vi "Auton - Center Shoot.vi"(10 "Alliance":T1, 11 "Auton States":T2=enum."Reset Encoders") -> ()   [LabVIEW 2016]
uses:
  Auton - Center Shoot States.ctl
  <vilib>/Rock Robotics/WPI/DriverStation/WPI_DriverStationAllianceInfo.ctl
  Robot Values.vi
panel:
  in  "Move To Boiler SP":dbl
  in  "Red - Turn  to Boiler SP":dbl
  in  "Blue - Turn  to Boiler SP":dbl
  in  "Move Toward Boiler SP":dbl
  in  "Red - Turn to Continue  SP":dbl format="%#_13g"
  in  "Blue - Turn to Continue  SP":dbl format="%#_13g"
  in  "Drive Off Wall SP":dbl
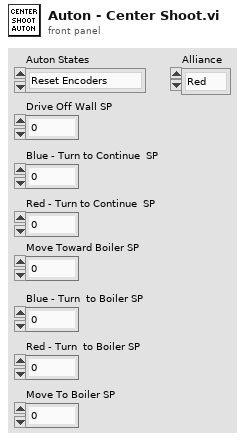
[diagram p1: front panel]
types:
  T1 = typedef "WPI_DriverStationAllianceInfo.ctl" = enum16{"Red", "Blue", "Invalid"}
  T2 = typedef "Auton - Center Shoot States.ctl" = enum16{"Stop", "Reset Encoders", "Drive Off Wall", "Turn to continue", "Reset Encoders Again", "Move toward Boiler", "Turn to Boiler", "Reset Encoders 3", "Move to Boiler", "Shoot"}
  T3 = typedef "Robot Values.ctl" = cluster{"Robot Drive":cluster{"Left Motor Power":dbl, "Right Motor Power":dbl, "Left Encoder Value":dbl, "Right Encoder Value":dbl, "High Gear?":bool, "PTO?":bool}, "Sensors":cluster{"Gyro Angle":u16, "Recalibrate Gyro":bool, "Reset Gyro":bool, "Ultrasonic":dbl}, "Shooter":cluster{"Prep Wheels":bool, "Shoot":bool, "Left Shooter Wheel Speed":dbl, "Wheels Moving":bool, "Shooter Prepped":bool, "Shooter RPS SP":dbl, "Shooting?":bool, "Left Shooter Wheel Power":dbl, "Right Shooter Wheel Power":dbl, "Acquisition Conveyor Power":dbl, "Hopper Beater Bar Power":dbl, "Filtered Left Shooter Speed":dbl, "Acquisition Motor Power":dbl, "Joystick Add":dbl, "D-Pad Add":dbl, "Shooter Use PID?":bool}, "Robot States":cluster{"Drive mode":string, "Alliance":T1, "Position":T4}, "Gear":cluster{"Ejection Active":bool}}
  T4 = typedef "WPI_DriverStationPositionInfo.ctl" = enum16{"1", "2", "3"}
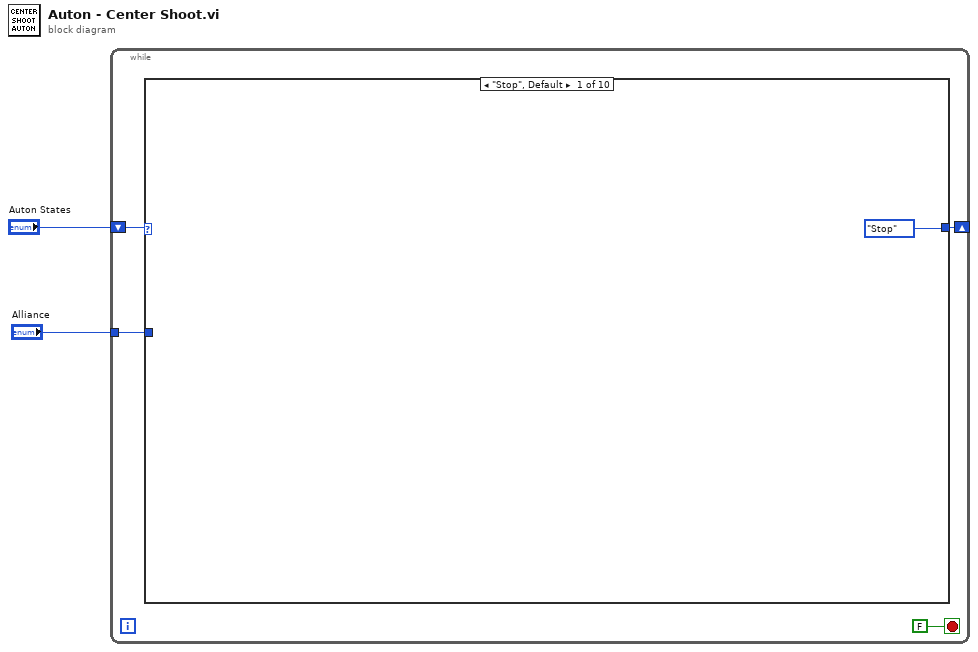
[diagram p0: block diagram]
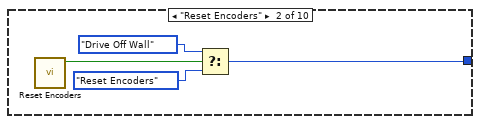
[diagram p2: hidden frame]
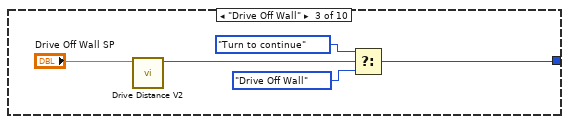
[diagram p3: hidden frame]
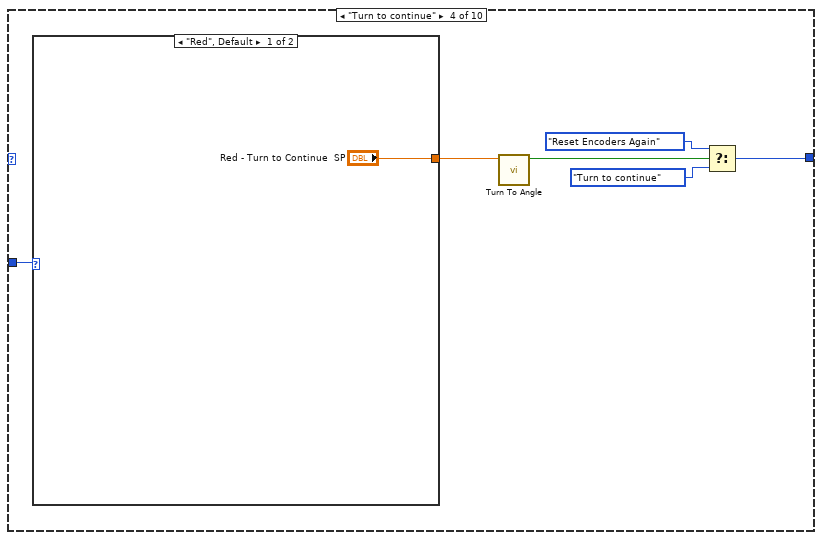
[diagram p4: hidden frame]
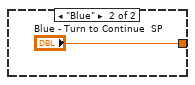
[diagram p5: hidden frame]
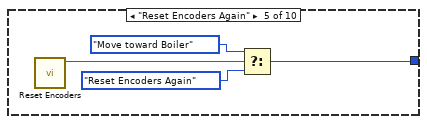
[diagram p6: hidden frame]
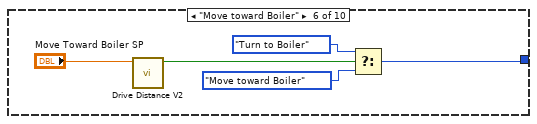
[diagram p7: hidden frame]
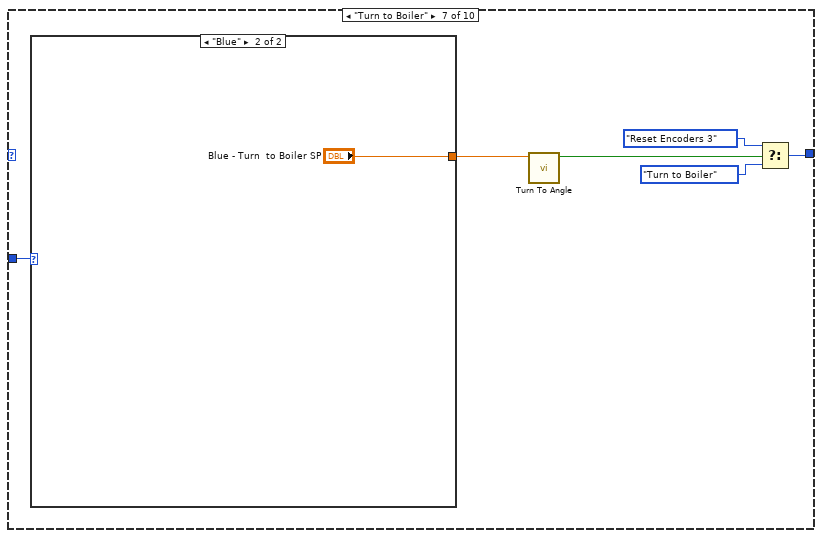
[diagram p8: hidden frame]
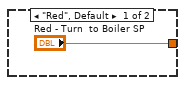
[diagram p9: hidden frame]
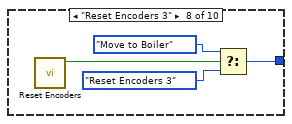
[diagram p10: hidden frame]
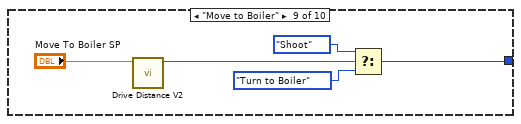
[diagram p11: hidden frame]
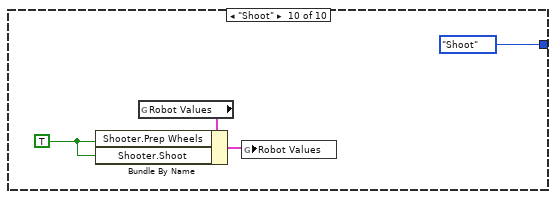
[diagram p12: hidden frame]
diagram:
  n1 = while {
    tunnel: "Alliance" -> [w5]
    shift-right: [w3] -> _
    shift-left: "Auton States" -> [w4]
    stop <- FALSE stop-if-true
    n2 = case shown="\"Stop\", Default" w4 {
      tunnel: w5 -> [_ _ _ w22 _ _ w39 _ _ _]
      tunnel: [Auton_-_Center_Shoot_States."Stop" ("Auton States 2") w9 w14 w19 w25 w29 w36 w42 w46 Auton_-_Center_Shoot_States."Shoot" ("Auton States 2")] -> w3
      frame "Stop", Default {
      }
      frame "Reset Encoders" {
        n3 = call "Reset Encoders.vi"() -> ("Done?"=w11:bool)  [unwired: 11 in]
        n4 = Select(t=Auton_-_Center_Shoot_States."Drive Off Wall" ("Auton States 2"), s=w11, f=Auton_-_Center_Shoot_States."Reset Encoders" ("Auton States 2")) -> (s? t:f=w9:T2)
      }
      frame "Drive Off Wall" {
        n5 = call "Drive Distance V2.vi"("Distance Set Point"="Drive Off Wall SP") -> ("Done?"=w13:bool)  [unwired: 10 in]
        n6 = Select(t=Auton_-_Center_Shoot_States."Turn to continue" ("Auton States 2"), s=w13, f=Auton_-_Center_Shoot_States."Drive Off Wall" ("Auton States 2")) -> (s? t:f=w14:T2)
      }
      frame "Turn to continue" {
        n7 = case shown="\"Red\", Default" w22 {
          tunnel: ["Red - Turn to Continue  SP" "Blue - Turn to Continue  SP"] -> w17
          frame "Red", Default {
          }
          frame "Blue" {
          }
        }
        n8 = call "Turn To Angle.vi"("Setpoint"=w17) -> ("Done?"=w18:bool)  [unwired: 10 in]
        n9 = Select(t=Auton_-_Center_Shoot_States."Reset Encoders Again" ("Auton States 2"), s=w18, f=Auton_-_Center_Shoot_States."Turn to continue" ("Auton States 2")) -> (s? t:f=w19:T2)
      }
      frame "Reset Encoders Again" {
        n10 = call "Reset Encoders.vi"() -> ("Done?"=w26:bool)  [unwired: 11 in]
        n11 = Select(t=Auton_-_Center_Shoot_States."Move toward Boiler" ("Auton States 2"), s=w26, f=Auton_-_Center_Shoot_States."Reset Encoders Again" ("Auton States 2")) -> (s? t:f=w25:T2)
      }
      frame "Move toward Boiler" {
        n12 = call "Drive Distance V2.vi"("Distance Set Point"="Move Toward Boiler SP") -> ("Done?"=w32:bool)  [unwired: 10 in]
        n13 = Select(t=Auton_-_Center_Shoot_States."Turn to Boiler" ("Auton States 2"), s=w32, f=Auton_-_Center_Shoot_States."Move toward Boiler" ("Auton States 2")) -> (s? t:f=w29:T2)
      }
      frame "Turn to Boiler" {
        n14 = case shown="\"Blue\"" w39 {
          tunnel: ["Red - Turn  to Boiler SP" "Blue - Turn  to Boiler SP"] -> w34
          frame "Red", Default {
          }
          frame "Blue" {
          }
        }
        n15 = call "Turn To Angle.vi"("Setpoint"=w34) -> ("Done?"=w35:bool)  [unwired: 10 in]
        n16 = Select(t=Auton_-_Center_Shoot_States."Reset Encoders 3" ("Auton States 2"), s=w35, f=Auton_-_Center_Shoot_States."Turn to Boiler" ("Auton States 2")) -> (s? t:f=w36:T2)
      }
      frame "Reset Encoders 3" {
        n17 = call "Reset Encoders.vi"() -> ("Done?"=w43:bool)  [unwired: 11 in]
        n18 = Select(t=Auton_-_Center_Shoot_States."Move to Boiler" ("Auton States 2"), s=w43, f=Auton_-_Center_Shoot_States."Reset Encoders 3" ("Auton States 2")) -> (s? t:f=w42:T2)
      }
      frame "Move to Boiler" {
        n19 = call "Drive Distance V2.vi"("Distance Set Point"="Move To Boiler SP") -> ("Done?"=w48:bool)  [unwired: 10 in]
        n20 = Select(t=Auton_-_Center_Shoot_States."Shoot" ("Auton States 2"), s=w48, f=Auton_-_Center_Shoot_States."Turn to Boiler" ("Auton States 2")) -> (s? t:f=w46:T2)
      }
      frame "Shoot" {
        w54 = TRUE
        n21 = global read "Robot Values.vi" "Robot Values"() -> (w52:T3)
        n22 = Bundle By Name(cluster=w52, "Shooter.Prep Wheels"=w54, "Shooter.Shoot"=w54) -> (w53:T3)
        n23 = global write "Robot Values.vi" "Robot Values"(w53) -> ()
      }
    }
  }
